vi "_Veritech_LVCM_Global_Init.vi"(11 "Object":T1) -> ()   [LabVIEW 2014]
uses:
  <resource>/Framework/Providers/API/ItemRef.ctl
  <resource>/Framework/Providers/API/mxLvMenuItem.ctl
  Support/Utilites/GCMLog/GCMLog.lvclass
panel:
  out "error out":errorcluster
  in  "error in":errorcluster
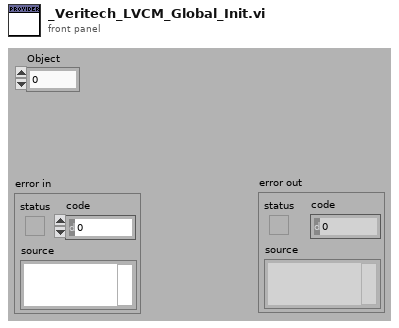
[diagram p1: front panel]
types:
  T1 = typedef "ItemRef.ctl" = u64
  T2 = typedef "mxLvMenuItem.ctl" = cluster{"Menu Name":string, "Description":string, "Icon File Name":path, "Menu Tag":string, "Enabled":bool, "Checked":bool, "Separator":bool, "Batchable":bool, "Weight":i32, "Batch Mode (Ignored if Not Batchable)":enum32{"Show If All Items Support Command", "Show If Any Items Support Command"}, "Menu Location":enum32{"<None>", "Project", "Project / Build Specifications", "Tools", "Tools / Source Control", "Tools / Real-Time Module", "Help"}, "Exclude From Getting Started Window Menu":bool}
  T3 = enum32{"<None>", "Project", "Project / Build Specifications", "Tools", "Tools / Source Control", "Tools / Real-Time Module", "Help"}
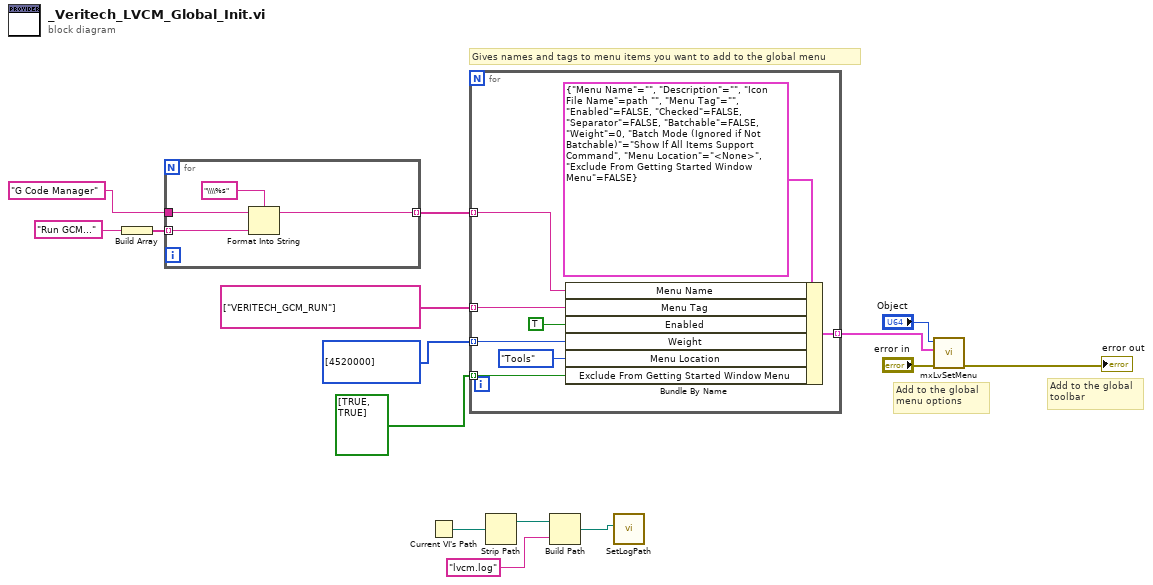
[diagram p0: block diagram]
diagram:
  # "Add to the global\ntoolbar"
  # "Add to the global\nmenu options"
  # "Gives names and tags to menu items you want to add to the global menu"
  n1 = Build Array("Run GCM..." ("SecondaryProviderExample1")) -> (w12:string[])
  n2 = for {
    tunnel: w12 -> [w16] mode=indexing
    tunnel: "G Code Manager" ("SecondaryProviderExample1") -> [w19]
    tunnel: [w18] -> w11 mode=indexing
    n3 = Format Into String(format string="\\\\%s", initial string=w19, w16) -> (resulting string=w18:string)  [unwired: 1 in, 1 out]
  }
  n4 = Current VI's Path() -> (path=w4:path)
  n5 = for {
    tunnel: [w27] -> w14 mode=indexing
    tunnel: i32[] [4520000] ("menu weight") -> [w26] mode=indexing
    tunnel: string[] ["VERITECH_GCM_RUN"] ("menu tag") -> [w25] mode=indexing
    tunnel: w11 -> [w23] mode=indexing
    tunnel: bool[] [TRUE, TRUE] ("exclude from GSW") -> [w24] mode=indexing
    n6 = Bundle By Name(cluster=T2 {"Menu Name"="", "Description"="", "Icon File Name"=path "", "Menu Tag"="", "Enabled"=FALSE, "Checked"=FALSE, "Separator"=FALSE, "Batchable"=FALSE, "Weight"=0, "Batch Mode (Ignored if Not Batchable)"=enum."Show If All Items Support Command", "Menu Location"=enum."<None>", "Exclude From Getting Started Window Menu"=FALSE} ("Menu Item"), "Menu Name"=w23, "Menu Tag"=w25, "Enabled"=TRUE ("Checked"), "Weight"=w26, "Menu Location"=T3."Tools", "Exclude From Getting Started Window Menu"=w24) -> (w27:T2)
  }
  n7 = Strip Path(path=w4) -> (stripped path=w3:path)  [unwired: 1 out]
  n8 = Build Path(base path=w3, name or relative path="lvcm.log") -> (appended path=w1:path)
  n9 = call "SetLogPath.vi"("LogPath"=w1) -> ()  [unwired: 10 in, 1 out]
  n10 = call <resource>:"mxLvSetMenu.vi"("error in"="error in", "Menu Items"=w14, "Item"="Object") -> ("error out"=→"error out":errorcluster)  [unwired: 8 out]
